vi "CFWSMetClient.vi"() -> (0 "Time Of Value (s)":dbl format="%#.1f", 1 "error out":errorcluster, 2 "RawPressure/mBar":dbl)   [LabVIEW 2016]
panel:
  out "ComputerTime":timestamp
  out "MetTimeStamp":timestamp
  out "data out":string
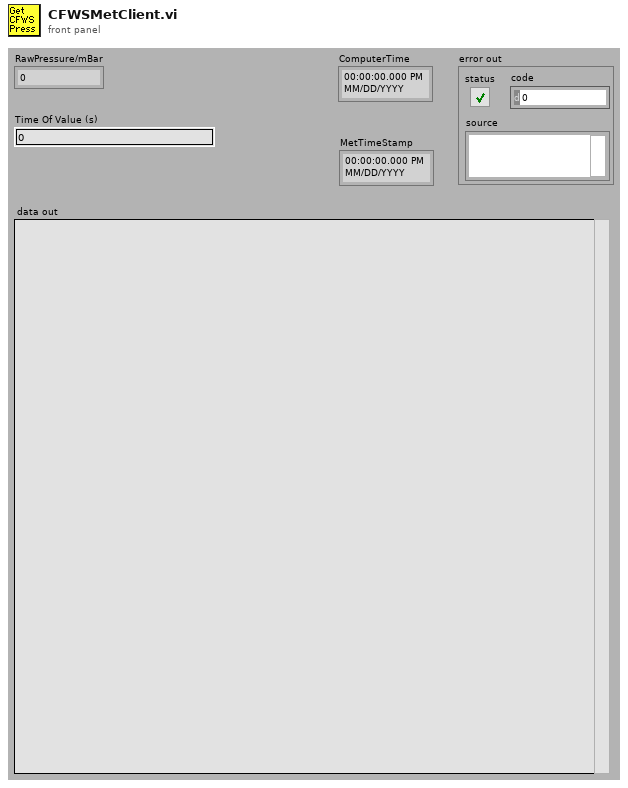
[diagram p1: front panel]
types:
  T1 = cluster{"second":i32, "minute":i32, "hour":i32, "day of month":i32, "month":i32, "year":i32, "day of week":i32, "day of year":i32, "is DST":i32}
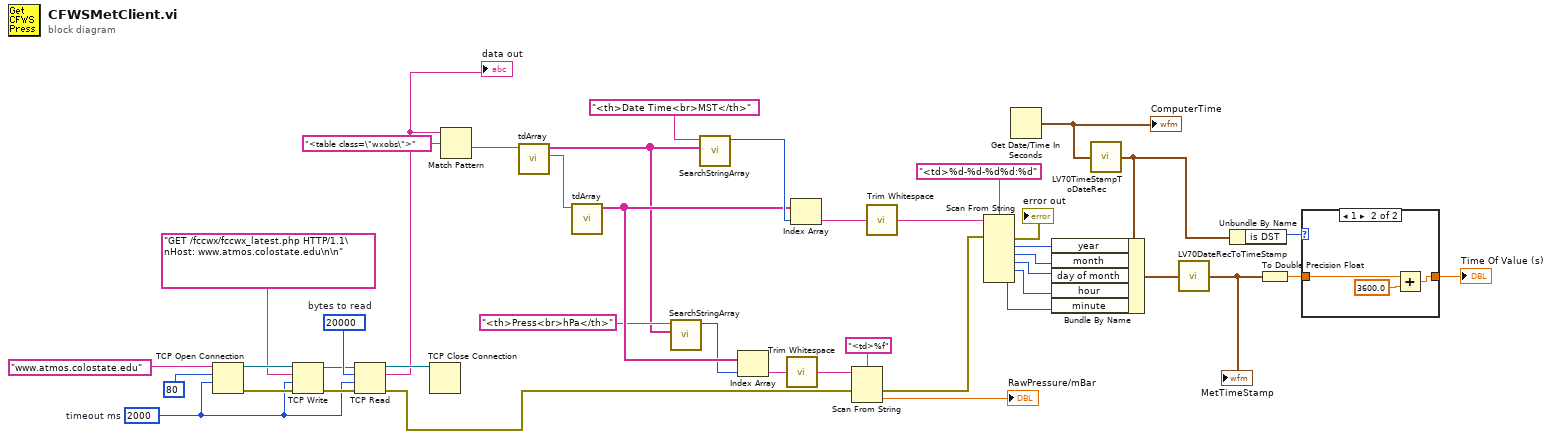
[diagram p0: block diagram]
diagram:
  w11 = 2000  # timeout ms
  w35 = 20000  # bytes to read
  n1 = TCP Open Connection(address="www.atmos.colostate.edu", remote port or service name=u16 80 ("remote port"), timeout ms (60000)=w11) -> (connection ID=w40:refnum<k5>, error out=w38:errorcluster)  [unwired: 1 in, 1 out]
  n2 = TCP Write(connection ID=w40, data in="GET /fccwx/fccwx_latest.php HTTP/1.1\nHost: www.atmos.colostate.edu\n\n", error in (no error)=w38, 9:w11) -> (connection ID out=w34:refnum<k5>, error out=w37:errorcluster)  [unwired: 1 out]
  n3 = TCP Read(connection ID=w34, bytes to read=w35, error in (no error)=w37, 9:w11) -> (connection ID out=w36:refnum<k5>, data out=w30:string, error out=w1:errorcluster)  [unwired: 1 out]
  "data out" <- w30
  n4 = TCP Close Connection(connection ID=w36) -> ()  [unwired: 1 in, 3 out]
  n5 = Match Pattern(string=w30, regular expression="<table class=\"wxobs\">") -> (after substring=w28:string)  [unwired: 4 out]
  n6 = call "tdArray.vi"("tableIn"=w28) -> ("remainingTable"=w8:string, "firstRow"=w5:string[])  [unwired: 9 in]
  n7 = call "tdArray.vi"("tableIn"=w8) -> ("firstRow"=w7:string[])  [unwired: 9 in, 1 out]
  n8 = call "SearchStringArray.vi"("stringArray"=w5, "String"="<th>Press<br>hPa</th>") -> ("foundIndex"=w4:i32)  [unwired: 9 in]
  n9 = call "SearchStringArray.vi"("stringArray"=w5, "String"="<th>Date Time<br>MST</th>") -> ("foundIndex"=w27:i32)  [unwired: 9 in]
  n10 = Index Array(array=w7, index=w4) -> (element=w15:string)
  n11 = call <vilib>:"Trim Whitespace.vi"("string"=w15) -> ("trimmed string"=w16:string)  [unwired: 1 in]
  n12 = Index Array(array=w7, index=w27) -> (element=w24:string)
  n13 = Scan From String(format string="<td>%f", input string=w16, error in=w1) -> (error out=w3:errorcluster, output 1=→"RawPressure/mBar":dbl)  [unwired: 1 in, 3 out]
  n14 = call <vilib>:"Trim Whitespace.vi"("string"=w24) -> ("trimmed string"=w17:string)  [unwired: 1 in]
  n15 = Scan From String(format string="<td>%d-%d-%d%d:%d", input string=w17, error in=w3) -> (error out=→"error out":errorcluster, output 1=w23:i32, output 2=w22:i32, output 3=w21:i32, output 4=w20:i32, output 5=w19:i32)  [unwired: 1 in, 7 out]
  n16 = Get Date/Time In Seconds() -> (seconds since 1Jan1904=w9:timestamp)
  "ComputerTime" <- w9
  n17 = call <vilib>:"LV70TimeStampToDateRec.vi"("time stamp"=w9) -> ("date time rec"=w12:T1)
  n18 = Bundle By Name(cluster=w12, "year"=w23, "month"=w22, "day of month"=w21, "hour"=w20, "minute"=w19) -> (w18:T1)
  n19 = call <vilib>:"LV70DateRecToTimeStamp.vi"("date time rec"=w18) -> ("Time Stamp"=w10:timestamp)
  "MetTimeStamp" <- w10
  n20 = Unbundle By Name(w12) -> ("is DST"=w33:i32)
  n21 = To Double Precision Float(number=w10) -> (double precision float=w32:dbl)
  n22 = case shown="1" w33 {
    tunnel: w32 -> [w43 w46]
    tunnel: [w43 w44] -> w31
    frame 0, Default {
    }
    frame 1 {
      n23 = Add(x=w46, y=3600.0) -> (x+y=w44:dbl)
    }
  }
  "Time Of Value (s)" <- w31
